vi "LuaVIEW Pull (path).vi"(5 "LuaVIEW reference in":T1, 11 "error in (no error)":errorcluster) -> (4 "path":path, 6 "LuaVIEW reference out":T1, 15 "error out":errorcluster)   [LabVIEW 2013]
doc: "Returns the path converted from a string at the head/bottom of the Lua stack. The string is subsequently removed, thereby shifting any remaining data items down by one. Beware that, if so configured, the string to path conversion might treat path seperators in a manner that differs slightly from LabVIEW's string to path conversion. Please refer to the manual appendix describing the various supported data types for details. This VI is part of a polymorphic set that supports the pulling various data types. To change the type being pulled, pop up on this VI's diagram icon and use the \"Select Type\" sub menu."
uses:
  typedefs/t_LuaVIEW Reference.ctl
  typedefs/et_LuaVIEW CIN Actions.ctl
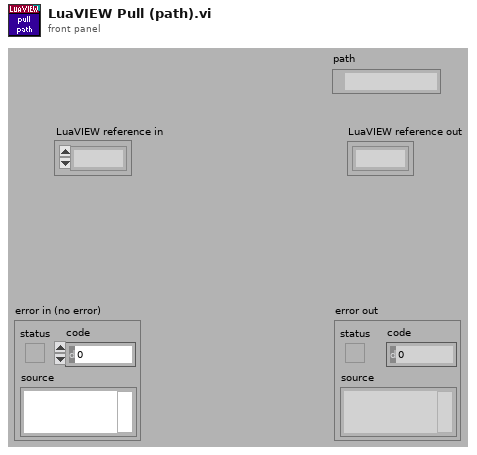
[diagram p1: front panel]
types:
  T1 = typedef "t_LuaVIEW Reference.ctl" = refnum<k1>
  T2 = typedef "et_LuaVIEW CIN Actions.ctl" = enum16{"checksynopsis", "_open", "_registerpublic", "_registerexport", "__never_an_error_result_ns", "luaversion", "cinversion", "_totals", "_taskcount", "pathological", "_unregnextpublic", "registryusecount", "__per_state_actions", "regsetprivate", "regsetindex", "regsetmodule", "_revokeexports", "_usepublic", "prepare", "compile", "execute", "call", "unregstaterefs", "_close", "pullboolean", "pullnumber", "pullI8", "pullU8", "pullI16", "pullU16", "pullI32", "pullU32", "pullobject", "pullrefnum", "pullstring", "pullflat", "pushflat", "pushobject", "getattribute", "setattribute", "stacktostring", "_startyieldtest", "_endyieldtest", "_pollprintbuffer", "__never_an_error_result_ps", "_pollexport", "setclone", "forcecleanup", "gettop", "clearstack", "insert", "pushboolean", "pushnumber", "pushrefnum", "pushstring", "pushnil", "pushvalue", "gettaskref", "settaskref"}
  T3 = typedef "et_LuaVIEW CIN Results.ctl" = enum16{"OK", "error", "main", "call", "clonecall", "modulecall", "exportcall", "index", "yield"}
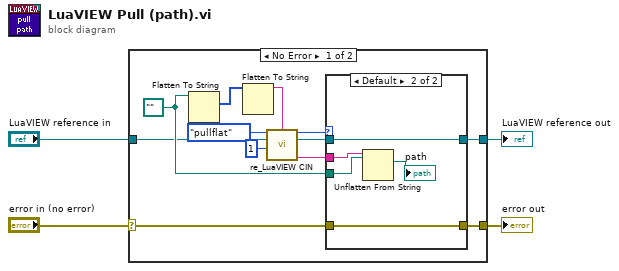
[diagram p0: block diagram]
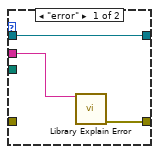
[diagram p2: hidden frame]
diagram:
  n1 = case shown="No Error" "error in (no error)" {
    selector: "error in (no error)" -> [w9 w26]
    tunnel: [w6 w25] -> w4
    tunnel: [w8 w26] -> w3
    tunnel: "LuaVIEW reference in" -> [w7 w25]
    frame No Error {
      w11 = path ""
      n2 = Flatten To String(anything=w11) -> (type string=w10:i16[])  [unwired: 3 in, 2 out]
      n3 = Flatten To String(anything=w10) -> (data string=w12:string)  [unwired: 3 in, 2 out]
      n4 = call "re_LuaVIEW CIN.vi"("action"=et_LuaVIEW_CIN_Actions."pullflat", "supplement"=w12, "LuaVIEW reference in"=w7, "index in"=1) -> ("result"=w14:T3, "LuaVIEW reference out"=w15:T1, "string out"=w13:string)  [unwired: 5 in, 4 out]
      n5 = case shown="Default" w14 {
        tunnel: w15 -> [w17 w23]
        tunnel: [w17 w23] -> w6
        tunnel: [w19 w24] -> w8
        tunnel: w13 -> [w18 w20]
        tunnel: w9 -> [_ w24]
        tunnel: w11 -> [_ w21]
        frame "error" {
          n6 = call "Library Explain Error.vi"("explanation prefix (none)"=w18) -> ("explained error"=w19:errorcluster)  [unwired: 14 in]
        }
        frame Default {
          n7 = Unflatten From String(type=w21, binary string=w20) -> (value=→"path":path)  [unwired: 3 in, 2 out]
        }
      }
    }
    frame Error {
    }
  }
  "LuaVIEW reference out" <- w4
  "error out" <- w3
